vi "Waveform Averager.vi"(1 "Samples to Average":i32, 2 "waveform":waveform(dbl)) -> (0 "output waveform":waveform(dbl))   [LabVIEW 2015]
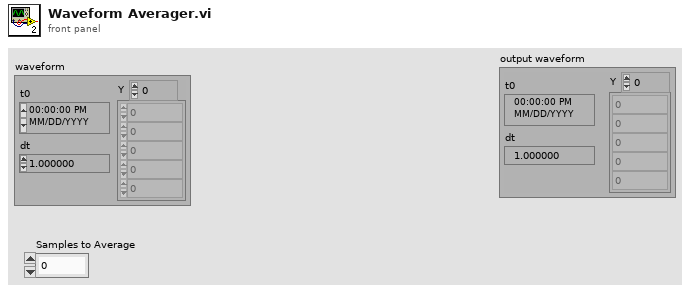
[diagram p1: front panel]
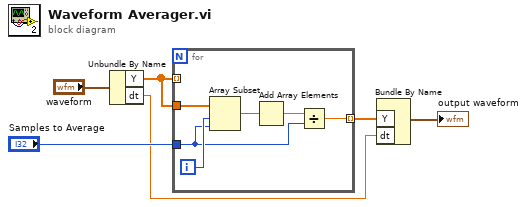
[diagram p0: block diagram]
diagram:
  n1 = Unbundle By Name("waveform") -> ("Y"=w6:dbl[], "dt"=w2:dbl)
  n2 = for {
    tunnel: w6 -> [_] mode=indexing
    tunnel: w6 -> [w12]
    tunnel: "Samples to Average" -> [w8]
    tunnel: [w7] -> w3 mode=indexing
    i -> [w11]
    n3 = Array Subset(array=w12, index=w11, length=w8) -> (w10:dbl[])
    n4 = Add Array Elements(numeric array=w10) -> (sum=w9:dbl)
    n5 = Divide(x=w9, y=w8) -> (x/y=w7:dbl)
  }
  n6 = Bundle By Name("Y"=w3, "dt"=w2) -> (→"output waveform":waveform(dbl))  [unwired: 1 in]
